vi "A系统时间.vi"() -> ()   [LabVIEW 2011]
uses:
  <vilib>/Utility/file.llb/Read From Spreadsheet File (string).vi
  <vilib>/Utility/file.llb/Write To Spreadsheet File (string).vi
panel:
  out "日期字符串":string
  in  "停止":bool
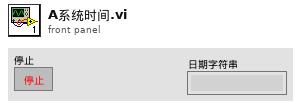
[diagram p1: front panel]
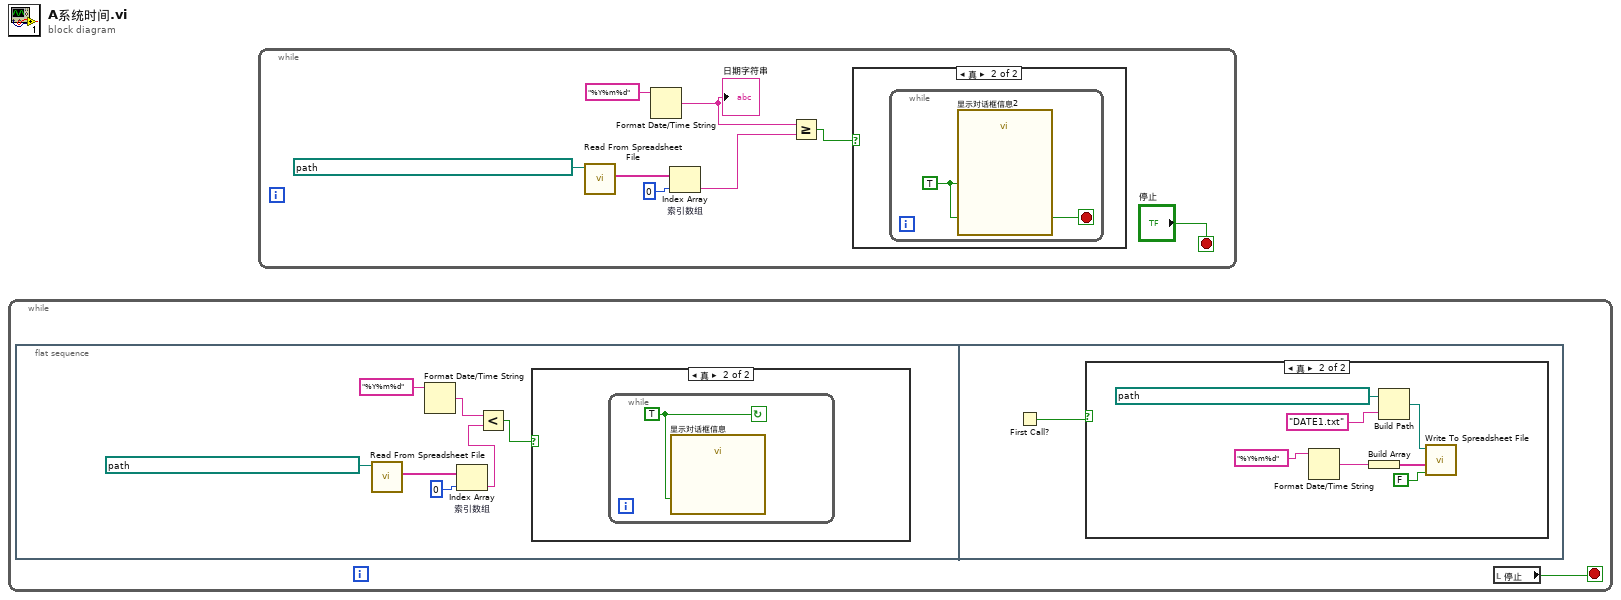
[diagram p0: block diagram]
diagram:
  n1 = while {
    stop <- w1 stop-if-true
    n2 = flat-sequence {
      frame #0 {
        n3 = call-poly <vilib>:"Read From Spreadsheet File.vi"("file path (dialog if empty)"=path "D:/程序/Q12012/B/人机界面/子VI/DATE1.txt") -> ("first row"=w5:string[])  [unwired: 6 in, 4 out]
        n4 = Format Date/Time String ("格式化日期/时间字符串")(time format string (%c)="%Y%m%d" ("时间格式字符串(%c)")) -> (date/time string=w3:string)  [unwired: 2 in]
        n5 = Index Array "索引数组"(array=w5, index=0 ("禁用的索引 (列)")) -> (element=w2:string)
        n6 = Less?(x=w3, y=w2) -> (x < y?=w4:bool)
        n7 = case shown="真" w4 {
          frame False {
          }
          frame True {
            n8 = while {
              stop <- w9 continue-if-true
              w9 = TRUE ("Enable")
              n9 = call "显示对话框信息"("Enable"=w9) -> ()  [unwired: 9 in, 2 out]
            }
          }
        }
      }
      frame #1 {
        n10 = First Call?() -> (First Call?: T/F=w10:bool)
        n11 = case shown="真" w10 {
          frame False {
          }
          frame True {
            n12 = Format Date/Time String ("格式化日期/时间字符串")(time format string (%c)="%Y%m%d" ("时间格式字符串(%c)")) -> (date/time string=w16:string)  [unwired: 2 in]
            n13 = Build Array(w16) -> (w15:string[])
            n14 = Build Path(base path=path "D:/程序/Q12012/B/人机界面/子VI/DATE1.txt" ("基路径"), name or relative path="DATE1.txt" ("名称或相对路径")) -> (appended path=w11:path)
            n15 = call-poly <vilib>:"Write To Spreadsheet File.vi"("append to file? (new file:F)"=FALSE, "1D data"=w15, "file path (dialog if empty)"=w11) -> ()  [unwired: 5 in, 1 out]
          }
        }
      }
    }
    n16 = local read "停止"() -> (w1:bool)
  }
  n17 = while {
    stop <- "停止" stop-if-true
    n18 = call-poly <vilib>:"Read From Spreadsheet File.vi"("file path (dialog if empty)"=path "D:/程序/Q12012/B/人机界面/子VI/DATE2.txt") -> ("first row"=w23:string[])  [unwired: 6 in, 4 out]
    n19 = Format Date/Time String ("格式化日期/时间字符串")(time format string (%c)="%Y%m%d" ("时间格式字符串(%c)")) -> (date/time string=w20:string)  [unwired: 2 in]
    "日期字符串" <- w20
    n20 = Index Array "索引数组"(array=w23, index=0 ("禁用的索引 (列)")) -> (element=w22:string)
    n21 = Greater Or Equal?(x=w20, y=w22) -> (x >= y?=w18:bool)
    n22 = case shown="真" w18 {
      frame False {
      }
      frame True {
        n23 = while {
          stop <- w26 stop-if-true
          w26 = TRUE ("Enable")
          n24 = call "显示对话框信息2"("Enable"=w26) -> ()  [unwired: 9 in, 2 out]
        }
      }
    }
  }
